vi "Read IK Recording Error File Write Cells.vi"(5 "Reason Column Letter":string="D", 7 "Depth Column Letter":string="C", 8 "error in (no error)":errorcluster, 9 "Row Offset In":i32, 10 "IK Recording Data file":path, 11 "NI_report in":refnum<class "NI_report.lvclass">) -> (0 "error out":errorcluster, 1 "all rows":string[][](array[string]), 2 "Row Offset Out":i32, 3 "NI_report out":refnum<class "NI_report.lvclass">)   [LabVIEW 2016]
uses:
  <vilib>/Utility/NIReport.llb/NI_report.lvclass
  <vilib>/Utility/file.llb/Read Delimited Spreadsheet (string).vi
panel:
  out "subarray":string[][](array[string])
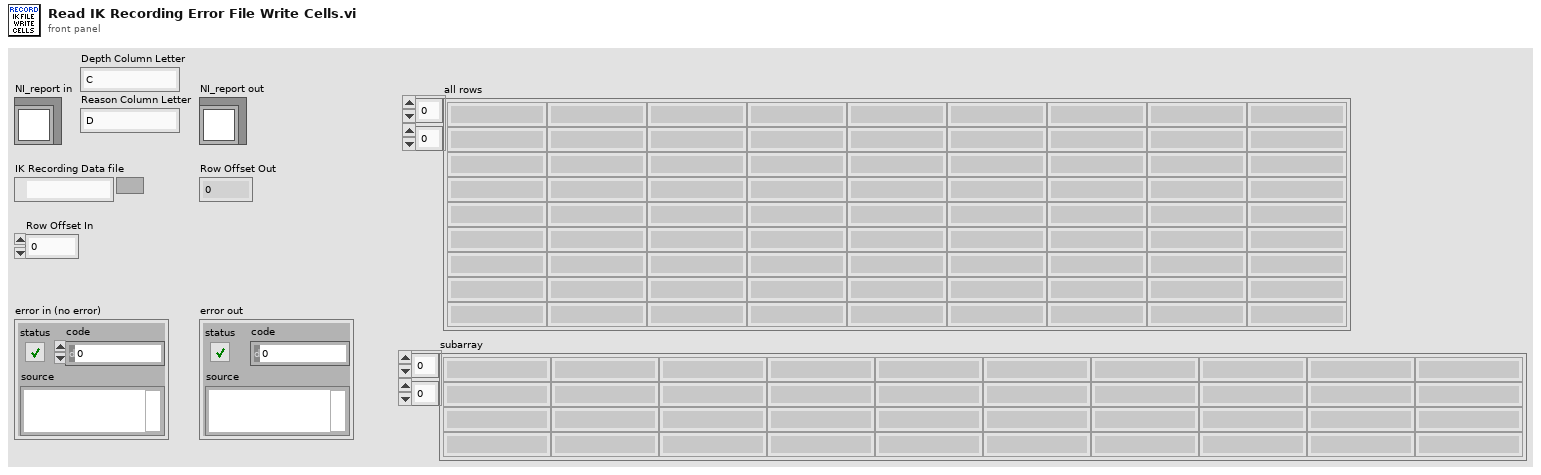
[diagram p1: front panel]
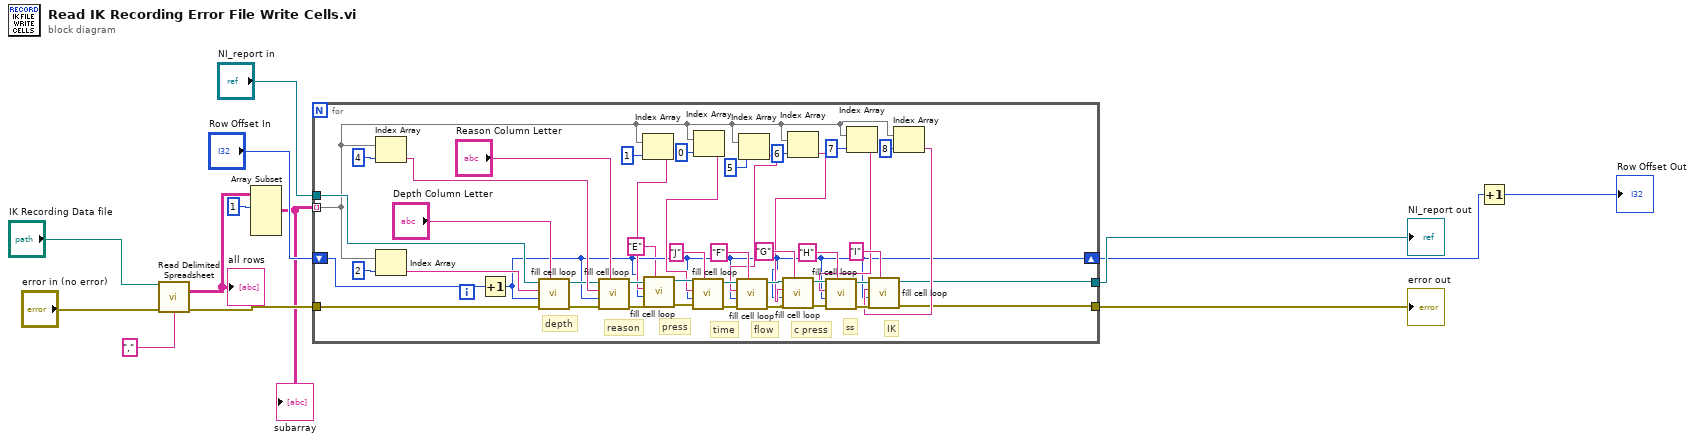
[diagram p0: block diagram]
diagram:
  n1 = call-poly <vilib>:"Read Delimited Spreadsheet.vi"("file path (dialog if empty)"="IK Recording Data file", "error in (no error)"="error in (no error)", "delimiter (\\t)"="," ("delimiter (\\t)")) -> ("all rows"=w4:string[][], "error out"=w13:errorcluster)  [unwired: 7 in, 4 out]
  "all rows" <- w4
  n2 = Array Subset(array=w4, index (row)=1 ("index")) -> (w6:string[][])  [unwired: 3 in]
  "subarray" <- w6
  n3 = for {
    tunnel: w6 -> [w20] mode=indexing
    shift-right: [w15] -> w9
    shift-left: "Row Offset In" -> [w58]
    tunnel: "NI_report in" -> [w50]
    tunnel: w13 -> [w53]
    tunnel: [w16] -> w11
    tunnel: [w17] -> w10
    # "IK"
    # "ss"
    # "c press"
    # "flow"
    # "time"
    # "press"
    # "reason"
    # "depth"
    n4 = Index Array(array=w20, index=4) -> (element=w54:string)
    n5 = Index Array(array=w20, index=2) -> (element=w51:string)
    n6 = Increment(x=w58) -> (x+1=w15:i32)
    n7 = call "fill cell loop.vi"("Column Letter"="Depth Column Letter", "error in (no error)"=w53, "Row"=w15, "String"=w51, "NI_report in"=w50) -> ("error out"=w52:errorcluster, "NI_report out"=w49:refnum<class "NI_report.lvclass">)  [unwired: 5 in]
    n8 = call "fill cell loop.vi"("Column Letter"="Reason Column Letter", "error in (no error)"=w52, "Row"=w15, "String"=w54, "NI_report in"=w49) -> ("error out"=w44:errorcluster, "NI_report out"=w45:refnum<class "NI_report.lvclass">)  [unwired: 5 in]
    n9 = Index Array(array=w20, index=1) -> (element=w34:string)
    n10 = call "fill cell loop.vi"("Column Letter"="E" ("String"), "error in (no error)"=w44, "Row"=w15, "String"=w34, "NI_report in"=w45) -> ("error out"=w47:errorcluster, "NI_report out"=w46:refnum<class "NI_report.lvclass">)  [unwired: 5 in]
    n11 = Index Array(array=w20, index=0) -> (element=w33:string)
    n12 = call "fill cell loop.vi"("Column Letter"="J", "error in (no error)"=w47, "Row"=w15, "String"=w33, "NI_report in"=w46) -> ("error out"=w42:errorcluster, "NI_report out"=w43:refnum<class "NI_report.lvclass">)  [unwired: 5 in]
    n13 = Index Array(array=w20, index=5) -> (element=w32:string)
    n14 = call "fill cell loop.vi"("Column Letter"="F", "error in (no error)"=w42, "Row"=w15, "String"=w32, "NI_report in"=w43) -> ("error out"=w40:errorcluster, "NI_report out"=w41:refnum<class "NI_report.lvclass">)  [unwired: 5 in]
    n15 = Index Array(array=w20, index=6) -> (element=w29:string)
    n16 = call "fill cell loop.vi"("Column Letter"="G", "error in (no error)"=w40, "Row"=w15, "String"=w29, "NI_report in"=w41) -> ("error out"=w28:errorcluster, "NI_report out"=w27:refnum<class "NI_report.lvclass">)  [unwired: 5 in]
    n17 = Index Array(array=w20, index=7) -> (element=w22:string)
    n18 = call "fill cell loop.vi"("Column Letter"="H", "error in (no error)"=w28, "Row"=w15, "String"=w22, "NI_report in"=w27) -> ("error out"=w26:errorcluster, "NI_report out"=w25:refnum<class "NI_report.lvclass">)  [unwired: 5 in]
    n19 = Index Array(array=w20, index=8) -> (element=w18:string)
    n20 = call "fill cell loop.vi"("Column Letter"="I", "error in (no error)"=w26, "Row"=w15, "String"=w18, "NI_report in"=w25) -> ("error out"=w16:errorcluster, "NI_report out"=w17:refnum<class "NI_report.lvclass">)  [unwired: 5 in]
  }
  "error out" <- w11
  "NI_report out" <- w10
  n21 = Increment(x=w9) -> (x+1=→"Row Offset Out":i32)
